vi "CORDIC.vi"(8 "rotate":bool, 9 "z":i32, 10 "y":i32 format="%x", 11 "x":i32 format="%x") -> (1 "z'":i32 format="%x", 2 "y'":i32 format="%x", 3 "x'":i32 format="%x")   [LabVIEW 2015]
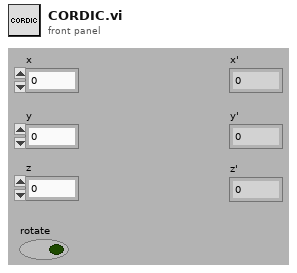
[diagram p1: front panel]
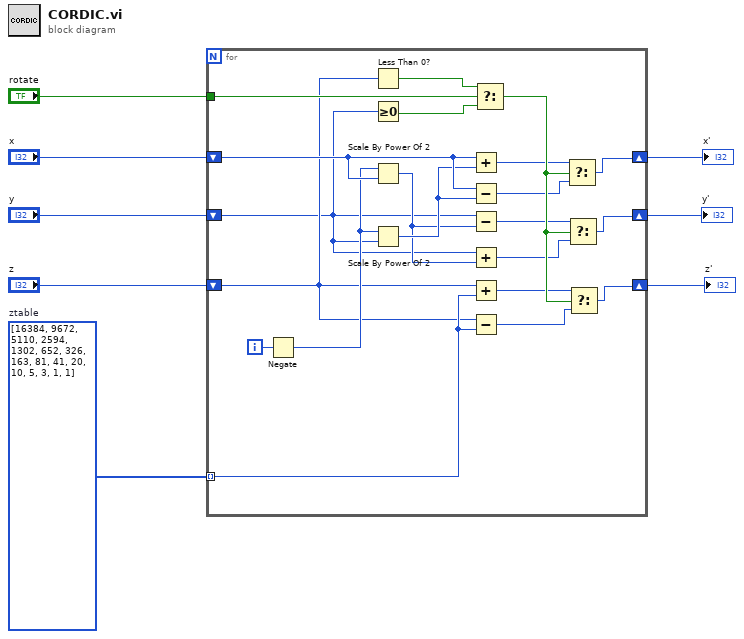
[diagram p0: block diagram]
diagram:
  w1 = i32[] [16384, 9672, 5110, 2594, 1302, 652, 326, 163, 81, 41, 20, 10, 5, 3, 1, 1]  # ztable
  n1 = for {
    tunnel: "rotate" -> [w29]
    shift-right: [w11] -> w8
    shift-left: "x" -> [w26]
    shift-right: [w10] -> w7
    shift-left: "y" -> [w12]
    shift-right: [w9] -> w2
    shift-left: "z" -> [w13]
    tunnel: w1 -> [w14] mode=indexing
    i -> [w18]
    n2 = Negate(x=w18) -> (-x=w15:i32)
    n3 = Less Than 0?(x=w13) -> (x < 0?=w28:bool)
    n4 = Greater Or Equal To 0?(x=w12) -> (x >= 0?=w27:bool)
    n5 = Scale By Power Of 2(n=w15, x=w26) -> (x*2^n=w20:i32)
    n6 = Scale By Power Of 2(n=w15, x=w12) -> (x*2^n=w23:i32)
    n7 = Add(x=w26, y=w23) -> (x+y=w22:i32)
    n8 = Subtract(x=w26, y=w23) -> (x-y=w24:i32)
    n9 = Subtract(x=w12, y=w20) -> (x-y=w21:i32)
    n10 = Add(x=w12, y=w20) -> (x+y=w19:i32)
    n11 = Add(x=w13, y=w14) -> (x+y=w17:i32)
    n12 = Subtract(x=w13, y=w14) -> (x-y=w16:i32)
    n13 = Select(t=w28, s=w29, f=w27) -> (s? t:f=w25:bool)
    n14 = Select(t=w22, s=w25, f=w24) -> (s? t:f=w11:i32)
    n15 = Select(t=w21, s=w25, f=w19) -> (s? t:f=w10:i32)
    n16 = Select(t=w17, s=w25, f=w16) -> (s? t:f=w9:i32)
  }
  "x'" <- w8
  "y'" <- w7
  "z'" <- w2
